vi "DRR_Query and display data.vi"(0 "System no.":i32=1 min=1 max=4 step=1, 2 "Rec. table IDs":i32[](array[numeric]), 3 "Without parameter?":bool, 5 "error in":errorcluster, 6 "Xo":i32=1, 7 "N":i32=100, 8 "Nmax":i32=1024) -> (14 "Data":dbl[][](array[numeric]) format="%.2f", 15 "Names":string[](array[string]), 16 "Sample Time":dbl format="%.10f", 19 "error out":errorcluster)   [LabVIEW 2020]
doc: "Returns N recorded data points and displays them in a 2D graph by calling Show_Save_Load_XY_Data.vi. N must be less than or equal to Nmax. For large N values, communication timeout must be set long enough, otherwise a comm.error may occur. If Sample time is zero, it is set to 1.0 for displaying data in the 2D graph only. \n\nAnalog: Rec. table IDs, x0, N and Nmax are not valid. Without parameter? must be TRUE.\n\nC-413: X0 >= 1. Nmax = 4096. The 4096 points are in equal shares assigned to the available data recorder tables. By default, the number of tables is 8. It can be reduced by setting the appropriate parameter value, see C-413 user manual for details.\n\nC-702: Nmax = 262144. X0 >= 0.\n\nC-843: X0 >= 1. Check C-843 user manual for valid Nmax values. Some hardware revisions don't allow the parallel use of DIO and the data recorder. To switch between both modes the C-843 needs to be reconnected. The number of tables is 4. The available points are in equal shares assigned to the available data recorder tables. By default, the number of tables is 4. It can be reduced with DRC, see C-843 user manual for details. If N = -1 all points of the last record are returned.\n\nC-866: X0 >= 1. Nmax = 32,256. If N = -1 all points of the last record are returned.\n\nC-867: X0 >= 1. Nmax = 8192. The number of tables is 4.\n\nC-877: Xo >= 1. Nmax = 8192.The number of tables is 4.\n\nC-884: Xo >= 1. Nmax = 8192. The number of tables is 8.\n\nC-891: Xo >= 1. Nmax = 16384.The C-891 has four data recorder tables with 4096 points per table. It can be changed to 1, 2 or 8 by setting the appropriate parameter value, see user manual for details.\n\nE-517, E-518: X0 >= 1. Nmax = 8192. The number of tables is 3.\n\nE-709: Xo >= 1. Nmax = 4096. The 4096 points are in equal shares assigned to the available data recorder tables. By default, the number of tables is 4. It can be reduced by setting the appropriate parameter value, see E-709 user manual for details.\n\nE-710: X0 >= 1. Nmax = 32,256.\n\nE-712: X0 >= 1. Nmax = 262,144. The 262,144 points are in equal shares assigned to the available data recorder tables. By default, the number of tables is 8. It can be reduced by setting the appropriate parameter value, see E-712 user manual for details.\n\nE-725, E-727: X0 >= 1. Nmax = 262,144. The 262,144 points are in equal shares assigned to the available data recorder tables. By default, the number of tables is 8. It can be reduced by setting the appropriate parameter value, see controller user manual for details. \n\nE-753: X0 >= 1. Nmax = 65,536. The 65,536 points are in equal shares assigned to the available data recorder tables. By default, the number of tables is 8. It can be reduced by setting the appropriate parameter value, see E-753 user manual for details.\n\nE-754: X0 >= 1. Nmax = 1,048,576. The 1,048,576 points are in equal shares assigned to the available data recorder tables. By default, the number of tables is 8. It can be reduced by setting the appropriate parameter value, see E-754 user manual for details.\n\nE-755: X0 >= 1. Nmax = 4,096.\n\nE-761: X0 >= 0. Recording takes place for all recorder tables as long as the wave generator is running for an arbitrary axis, when an impulse is started with IMP or when a step is started with STE. The assignment of axis and data sources to the recorder tables is as follows:\ntable 1: axis 1 actual position\ntable 2: axis 2 actual position\ntable 3: axis 3 actual position\ntable 4: analog input voltage (same value as read with TAV?, i.e. contains gain and offset for the analog input, see E-761 user manual).\nThe maximum number of data points is 8192 per recorder table.\n\nE-861: X0 >= 1. Nmax = 1024. Two data recorder tables with 1024 points per table are provided.\n\nE-871, E-873, E-874: Xo >= 1. Nmax = 1024. The number of tables is 2.\n\nC-887, F-206: Xo >= 1. See C-887 user manual for Nmax default value (can be changed with SPA.vi). Only for GCS syntax version = GCS 2.0 or higher (check with CSV?.vi. If CSV?.vi is not supported, syntax version is GCS 1.0). See controller user manual for available data recorder tables and points.\n\nC-887, M-8X0: For GCS syntax version = 1.0 (Check with CSV?.vi. If CSV?.vi is not supported, syntax version is GCS 1.0), Rec. table IDs, xo, N and Nmax are not valid and Without parameter? must be TRUE. \nFor GCS syntax version = 2.0, Xo >= 1. See C-887 user manual for Nmax default value (can be changed with SPA.vi).\nOnly supported if controller is based on C-842.80 board or GCS syntax version = GCS 2.0 or higher (Check with CSV?.vi. If CSV?.vi is not supported, syntax version is GCS 1.0). For GCS 1.0, returns 360 motor current values recorded during execution of DRV. \nFor GCS 2.0 and higher, see controller user manual for available data recorder tables and points. \n\nMercury_GCS: Xo >= 1. Nmax = 1024. See controller user manual for available data recorder tables."
panel:
  # "Returns N recorded data points and displays them in a 2D graph by calling \"Show_Save_Load_\nXY_Data.vi. N must be less than or equal to Nmax. For large N values, communication timeout \nmust be set long enough, otherwise a comm.error may occur."
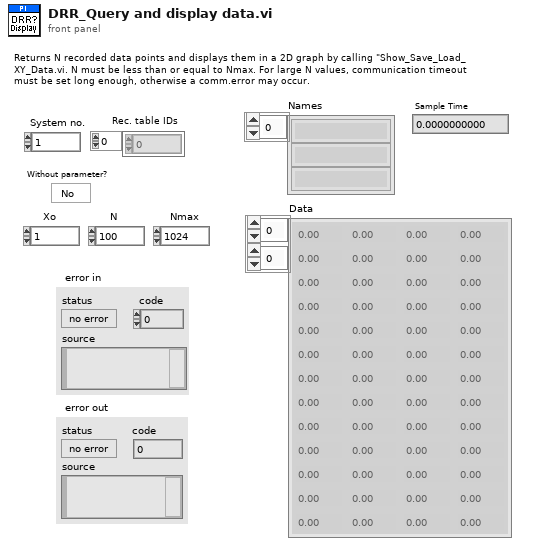
[diagram p1: front panel]
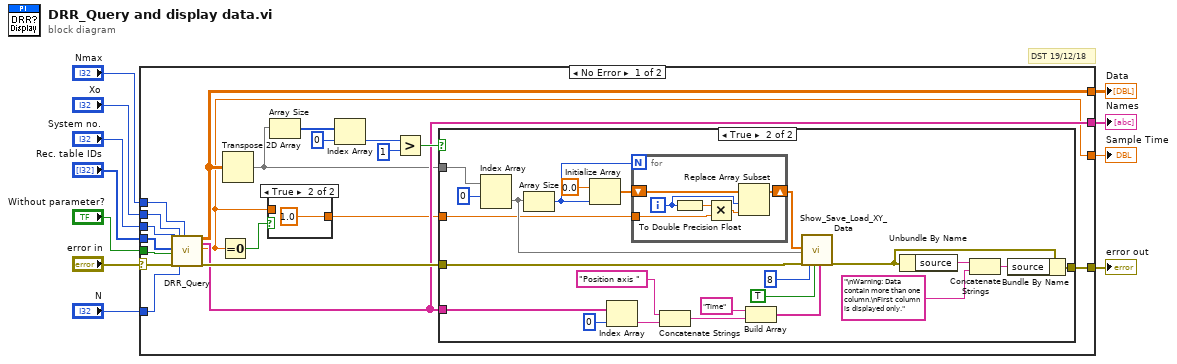
[diagram p0: block diagram]
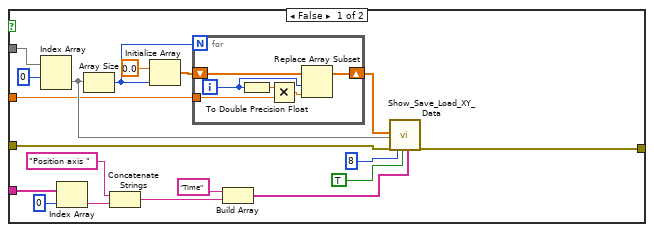
[diagram p3: hidden frame]
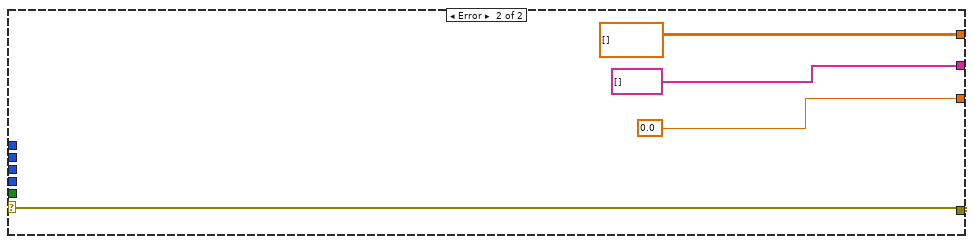
[diagram p4: hidden frame]
diagram:
  # "DST 19/12/18"
  n1 = case shown="No Error" "error in" {
    selector: "error in" -> [w12 w88]
    tunnel: "System no." -> [w31 _]
    tunnel: "Rec. table IDs" -> [w30 _]
    tunnel: [w25 w88] -> w10
    tunnel: [w18 dbl[][] [] ("Table out")] -> w6
    tunnel: "N" -> [w27 _]
    tunnel: "Xo" -> [w29 _]
    tunnel: "Nmax" -> [w28 _]
    tunnel: [w14 0.0 ("Sample Time out")] -> w5
    tunnel: [w19 string[] [] ("Names out")] -> w4
    tunnel: "Without parameter?" -> [w16 _]
    frame No Error {
      n2 = call "DRR_Query.vi"("System no."=w31, "Rec. table IDs"=w30, "Without parameter?"=w16, "error in"=w12, "Xo"=w29, "N"=w27, "Nmax"=w28) -> ("Data"=w18:dbl[][], "Names"=w19:string[], "Sample Time"=w14:dbl, "error out"=w26:errorcluster)  [unwired: 1 in, 8 out]
      n3 = Equal To 0?(x=w14) -> (x = 0?=w15:bool)
      n4 = Transpose 2D Array(2D array=w18) -> (transposed array=w17:dbl[][])
      n5 = case shown="True" w15 {
        tunnel: w14 -> [w32 _]
        tunnel: [w32 1.0 ("Sample Time")] -> w13
        frame False {
        }
        frame True {
        }
      }
      n6 = Array Size(array=w17) -> (size(s)=w24:i32[])
      n7 = Index Array(array=w24, index=0) -> (element=w22:i32)
      n8 = Greater?(x=w22, y=1) -> (0:w20:bool)
      n9 = case shown="True" w20 {
        tunnel: w17 -> [w46 w75]
        tunnel: w13 -> [w43 w72]
        tunnel: w26 -> [w42 w71]
        tunnel: [w41 w63] -> w25
        tunnel: w19 -> [w40 w70]
        frame False {
          n10 = Index Array(array=w46, index (row)=0) -> (element=w45:dbl[])  [unwired: 1 in]
          n11 = Index Array(array=w40, index=0) -> (element=w38:string)
          n12 = Array Size(array=w45) -> (size(s)=w52:i32)
          n13 = Concatenate Strings("Position axis " ("string"), w38) -> (w36:string)
          n14 = Initialize Array(0.0, w52) -> (w50:dbl[])
          n15 = for {
            N: w52 -> [_]
            shift-right: [w57] -> w49
            shift-left: w50 -> [w58]
            tunnel: w43 -> [w54]
            i -> [w55]
            n16 = To Double Precision Float(number=w55) -> (double precision float=w53:dbl)
            n17 = Multiply(x=w53, y=w54) -> (x*y=w56:dbl)
            n18 = Replace Array Subset(array=w58, new element=w56, index=w55) -> (w57:dbl[])
          }
          n19 = Build Array("Time" ("element"), w36) -> (w34:string[])
          n20 = call "Show_Save_Load_XY_Data.vi"("1D Array X"=w49, "1D Array Y"=w45, "error in"=w42, "No. of digits Y"=i16 8, "Autoscale"=TRUE, "Names"=w34) -> ("error out"=w41:errorcluster)  [unwired: 2 in, 11 out]
        }
        frame True {
          n21 = Index Array(array=w75, index (row)=0) -> (element=w74:dbl[])  [unwired: 1 in]
          n22 = Array Size(array=w74) -> (size(s)=w81:i32)
          n23 = Initialize Array(0.0, w81) -> (w79:dbl[])
          n24 = Index Array(array=w70, index=0) -> (element=w68:string)
          n25 = for {
            N: w81 -> [_]
            shift-right: [w86] -> w78
            shift-left: w79 -> [w87]
            tunnel: w72 -> [w83]
            i -> [w84]
            n26 = To Double Precision Float(number=w84) -> (double precision float=w82:dbl)
            n27 = Multiply(x=w82, y=w83) -> (x*y=w85:dbl)
            n28 = Replace Array Subset(array=w87, new element=w85, index=w84) -> (w86:dbl[])
          }
          n29 = Concatenate Strings("Position axis " ("string"), w68) -> (w66:string)
          n30 = Build Array("Time" ("element"), w66) -> (w64:string[])
          n31 = call "Show_Save_Load_XY_Data.vi"("1D Array X"=w78, "1D Array Y"=w74, "error in"=w71, "No. of digits Y"=i16 8, "Autoscale"=TRUE, "Names"=w64) -> ("error out"=w60:errorcluster)  [unwired: 2 in, 11 out]
          n32 = Unbundle By Name(w60) -> ("source"=w59:string)
          n33 = Concatenate Strings(w59, "\nWarning: Data contain more than one column.\nFirst column is displayed only." ("source")) -> (w61:string)
          n34 = Bundle By Name(cluster=w60, "source"=w61) -> (w63:errorcluster)
        }
      }
    }
    frame Error {
    }
  }
  "error out" <- w10
  "Data" <- w6
  "Sample Time" <- w5
  "Names" <- w4
